vi "createHPs.vi"(8 "error in (no error)":errorcluster, 11 "Boot in":refnum<class "Boot.lvclass">) -> (0 "error out":errorcluster, 2 "HPs":refnum<class "HPILC.lvclass">[](array[class]), 3 "Boot out":refnum<class "Boot.lvclass">)   [LabVIEW 2016, in "Boot.lvclass"]
uses:
  Boot.lvclass
  Common_RT_HPILC/HPILC/HPILC.lvclass
  Common_RT_HPILC/HPILCFactory/HPILCFactory.lvclass
  Common_RT_HPILC/DataTypes/HPSettings.ctl
  Common_RT_ILC/DataTypes/ILCSettings.ctl
  Common_RT_ILC/RTILC.lvlib
  Common_RT_HPILC/RTHPILC.lvlib
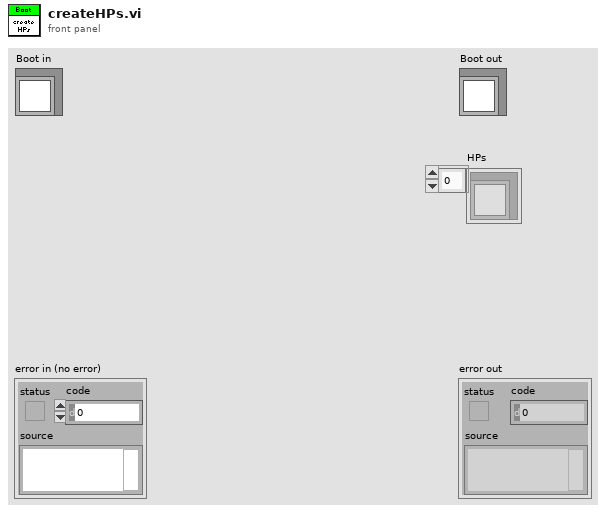
[diagram p1: front panel]
types:
  T1 = typedef "M1M3SupportSettings.lvlib/BaseILCSettings.ctl" = cluster{"CommunicationTimings":T2}
  T2 = typedef "RTILC.lvlib/ILCTimings.ctl" = cluster{"ADCOffsetSensitivity":u32, "ADCScanRate":u32, "ILCMode":u32, "ReadCalibration":u32, "ReportServerID":u32, "ReportServerStatus":u32, "Reset":u32, "SetTemporaryAddress":u32}
  T3 = typedef "M1M3SupportSettings.lvlib/BaseHPSettings.ctl" = cluster{"Identification":T4[], "CommunicationTimings":T5, "Positions":T6[]}
  T4 = typedef "M1M3SupportSettings.lvlib/BaseILCIdentitySettings.ctl" = cluster{"Subnet":u8, "Address":u8, "ID":i16}
  T5 = typedef "RTHPILC.lvlib/HPTimings.ctl" = cluster{"BroadcastStepMotor":u32, "ForceAndStatus":u32, "FreezeSensorValues":u32, "StepMotor":u32}
  T6 = typedef "M1M3SupportGeneral.lvlib/XYZPosition.ctl" = cluster{"X":sgl, "Y":sgl, "Z":sgl}
  T7 = typedef "M1M3SupportSettings.lvlib/HPSettings.ctl" = cluster{"ReferencePositions":i32[]}
  T8 = typedef "RTHPILC.lvlib/HPSettings.ctl" = cluster{"ILCSettings":T9, "ID":i16, "ReferencePosition":i32, "XPosition":sgl, "YPosition":sgl, "ZPosition":sgl}
  T9 = typedef "RTILC.lvlib/ILCSettings.ctl" = cluster{"Subnet":u8, "Address":u8}
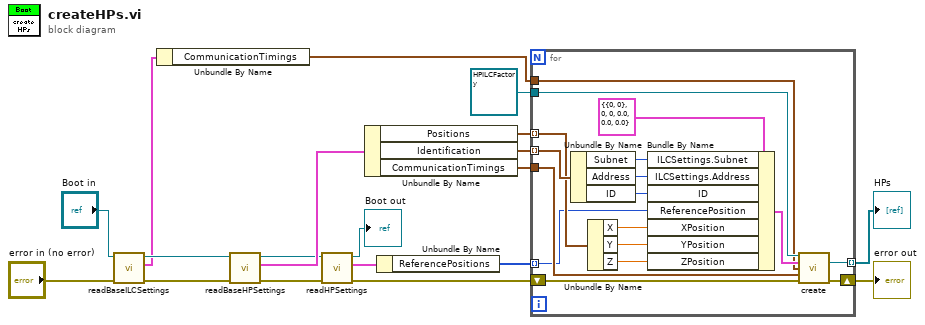
[diagram p0: block diagram]
diagram:
  n1 = call "readBaseILCSettings.vi"("error in (no error)"="error in (no error)", "Boot in"="Boot in") -> ("error out"=w10:errorcluster, "BaseHardpointSettings"=w9:T1, "Boot out"=w12:refnum<class "Boot.lvclass">)  [unwired: 7 in]
  n2 = Unbundle By Name(w9) -> ("CommunicationTimings"=w8:T2)
  n3 = call "readBaseHPSettings.vi"("error in (no error)"=w10, "Boot in"=w12) -> ("error out"=w5:errorcluster, "BaseHardpointSettings"=w19:T3, "Boot out"=w6:refnum<class "Boot.lvclass">)  [unwired: 7 in]
  n4 = call "readHPSettings.vi"("error in (no error)"=w5, "Boot in"=w6) -> ("error out"=w4:errorcluster, "HPSettings"=w2:T7, "Boot out"=→"Boot out":refnum<class "Boot.lvclass">)  [unwired: 7 in]
  n5 = Unbundle By Name(w19) -> ("Positions"=w7:T6[], "Identification"=w18:T4[], "CommunicationTimings"=w14:T5)
  n6 = Unbundle By Name(w2) -> ("ReferencePositions"=w1:i32[])
  n7 = for {
    tunnel: w18 -> [w36] mode=indexing
    tunnel: refnum<class "HPILCFactory.lvclass"> refnum ("RTHPILC.lvlib:HPILCFactory.lvclass") -> [w31]
    tunnel: [w29] -> w16 mode=indexing
    shift-right: [w27] -> w15
    shift-left: w4 -> [w28]
    tunnel: w14 -> [w26]
    tunnel: w8 -> [w25]
    tunnel: w7 -> [w24] mode=indexing
    tunnel: w1 -> [w20] mode=indexing
    n8 = Unbundle By Name(w36) -> ("Subnet"=w34:u8, "Address"=w33:u8, "ID"=w32:i16)
    n9 = Unbundle By Name(w24) -> ("X"=w23:sgl, "Y"=w22:sgl, "Z"=w21:sgl)
    n10 = Bundle By Name(cluster=T8 {"ILCSettings"={"Subnet"=0, "Address"=0}, "ID"=0, "ReferencePosition"=0, "XPosition"=0.0, "YPosition"=0.0, "ZPosition"=0.0} ("HPSettings"), "ILCSettings.Subnet"=w34, "ILCSettings.Address"=w33, "ID"=w32, "ReferencePosition"=w20, "XPosition"=w23, "YPosition"=w22, "ZPosition"=w21) -> (w30:T8)
    n11 = call "create.vi"("HPILCFactory in"=w31, "HPSettings"=w30, "ILCTimings"=w25, "HPTimings"=w26, "error in (no error)"=w28) -> ("HPILC"=w29:refnum<class "HPILC.lvclass">, "error out"=w27:errorcluster)  [unwired: 8 in, 1 out]
  }
  "error out" <- w15
  "HPs" <- w16
